vi "Com Port method.vi"() -> ()   [LabVIEW 2025]
uses:
  <vilib>/Instr/_visa.llb/VISA Configure Serial Port (Instr).vi
panel:
  in  "VISA resource name":refnum<visa-resource-name>
  out "error out 2":errorcluster
  in  "stop":bool
  out "Answer request main temperature area":string
  out "error out":errorcluster
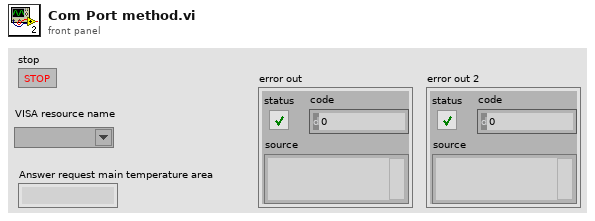
[diagram p1: front panel]
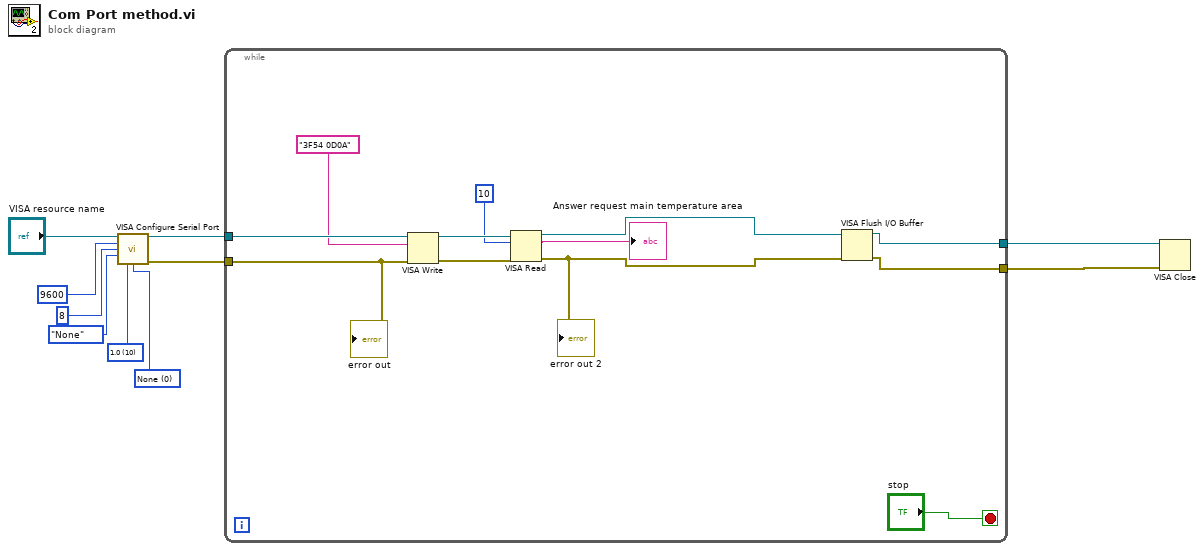
[diagram p0: block diagram]
diagram:
  w1 = u16 0 items=["None", "XON/XOFF", "RTS/CTS", "XON/XOFF & RTS/CTS", "DTR/DSR", "XON/XOFF & DTR/DSR"] ("flow control (0:none)")
  w2 = u16 10 items=["1.0"=10, "1.5"=15, "2.0"=20] ("stop bits (10: 1 bit)")
  n1 = call-poly "VISA Configure Serial Port"("VISA resource name"="VISA resource name", "baud rate (9600)"=u32 9600, "data bits (8)"=u16 8, "parity (0:none)"=enum16{"None", "Odd", "Even", "Mark", "Space"}."None", "stop bits (10: 1 bit)"=w2, "flow control (0:none)"=w1) -> ("VISA resource name out"=w10:refnum<visa-resource-name>, "error out"=w9:errorcluster)  [unwired: 8 in]
  n2 = while {
    tunnel: w10 -> [w22]
    tunnel: w9 -> [w21]
    tunnel: [w15] -> w8
    tunnel: [w13] -> w7
    stop <- "stop" stop-if-true
    n3 = VISA Write(VISA resource name=w22, write buffer="3F54 0D0A", error in (no error)=w21) -> (VISA resource name out=w18:refnum<visa-resource-name>, error out=w19:errorcluster)  [unwired: 1 out]
    n4 = VISA Read(VISA resource name=w18, byte count=u32 10, error in (no error)=w19) -> (VISA resource name out=w14:refnum<visa-resource-name>, read buffer=→"Answer request main temperature area":string, error out=w11:errorcluster)  [unwired: 1 out]
    "error out 2" <- w11
    n5 = VISA Flush I/O Buffer(VISA resource name=w14, error in (no error)=w11) -> (VISA resource name out=w13:refnum<visa-resource-name>, error out=w15:errorcluster)  [unwired: 1 in]
    "error out" <- w21
  }
  n6 = VISA Close(VISA resource name=w7, error in (no error)=w8) -> ()  [unwired: 1 out]
